vi "XY to Theta (2D picture).vi"(1 "y":dbl, 2 "x":dbl) -> (0 "Theta":dbl)   [LabVIEW 2021]
doc: "Range = [0,2pi)"
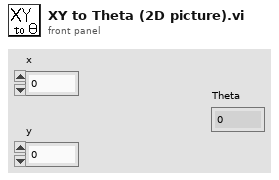
[diagram p1: front panel]
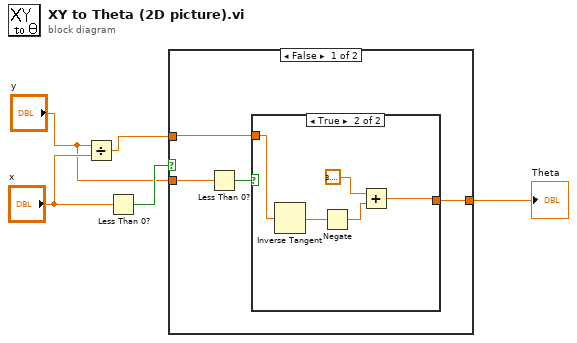
[diagram p0: block diagram]
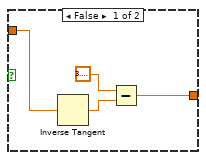
[diagram p2: hidden frame]
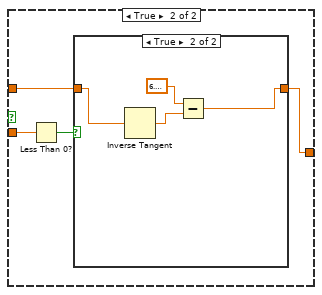
[diagram p3: hidden frame]
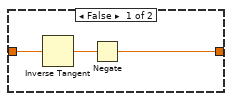
[diagram p4: hidden frame]
diagram:
  n1 = Divide(x="y", y="x") -> (x/y=w3:dbl)
  n2 = Less Than 0?(x="x") -> (x < 0?=w5:bool)
  n3 = case shown="False" w5 {
    tunnel: w3 -> [w7 w20]
    tunnel: "y" -> [w8 w21]
    tunnel: [w6 w19] -> w1
    frame False {
      n4 = Less Than 0?(x=w8) -> (x < 0?=w9:bool)
      n5 = case shown="True" w9 {
        tunnel: w7 -> [w11 w17]
        tunnel: [w10 w16] -> w6
        frame False {
          n6 = Inverse Tangent(1:w11) -> (0:w13:dbl)
          n7 = Subtract(x=3.141592653589793, y=w13) -> (x-y=w10:dbl)
        }
        frame True {
          n8 = Inverse Tangent(1:w17) -> (0:w14:dbl)
          n9 = Negate(x=w14) -> (-x=w15:dbl)
          n10 = Add(x=3.141592653589793, y=w15) -> (x+y=w16:dbl)
        }
      }
    }
    frame True {
      n11 = Less Than 0?(x=w21) -> (x < 0?=w22:bool)
      n12 = case shown="True" w22 {
        tunnel: w20 -> [w25 w28]
        tunnel: [w23 w26] -> w19
        frame False {
          n13 = Inverse Tangent(1:w25) -> (0:w24:dbl)
          n14 = Negate(x=w24) -> (-x=w23:dbl)
        }
        frame True {
          n15 = Inverse Tangent(1:w28) -> (0:w29:dbl)
          n16 = Subtract(x=6.283185307179586, y=w29) -> (x-y=w26:dbl)
        }
      }
    }
  }
  "Theta" <- w1
